vi "configurePerChannel.vi"(8 "error in (no error)":errorcluster, 10 "physical channels":string, 11 "K2602 in":refnum<class "K2602.lvclass">) -> (0 "error out":errorcluster, 3 "K2602 out":refnum<class "K2602.lvclass">)   [LabVIEW 2009, in "Hardware.lvlib" / "Channels.lvlib" / "K2602.lvclass"]
uses:
  K2602.lvclass
  K2602.lvclass/K2602.ctl
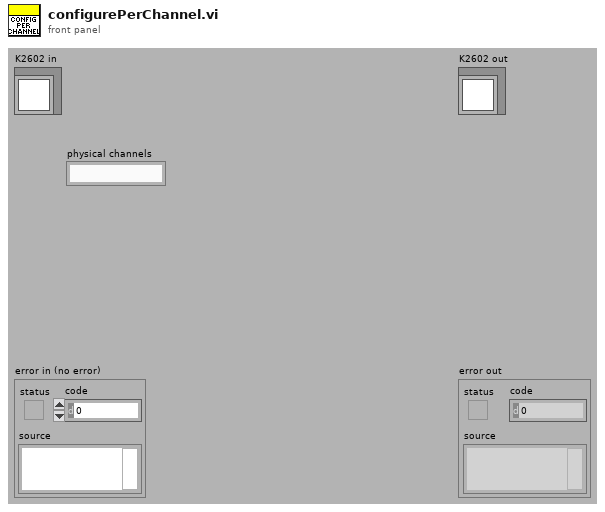
[diagram p1: front panel]
types:
  T1 = cluster{"Range":cluster{"current":dbl, "voltage":dbl}, "triggering_inUse":cluster{"start_trigger":string, "clock":string}, "Limits":cluster{"VoltageLimit":dbl, "CurrentLimit":dbl}}[]
  T2 = cluster{"Range":cluster{"current":dbl, "voltage":dbl}, "triggering_inUse":cluster{"start_trigger":string, "clock":string}, "Limits":cluster{"VoltageLimit":dbl, "CurrentLimit":dbl}}
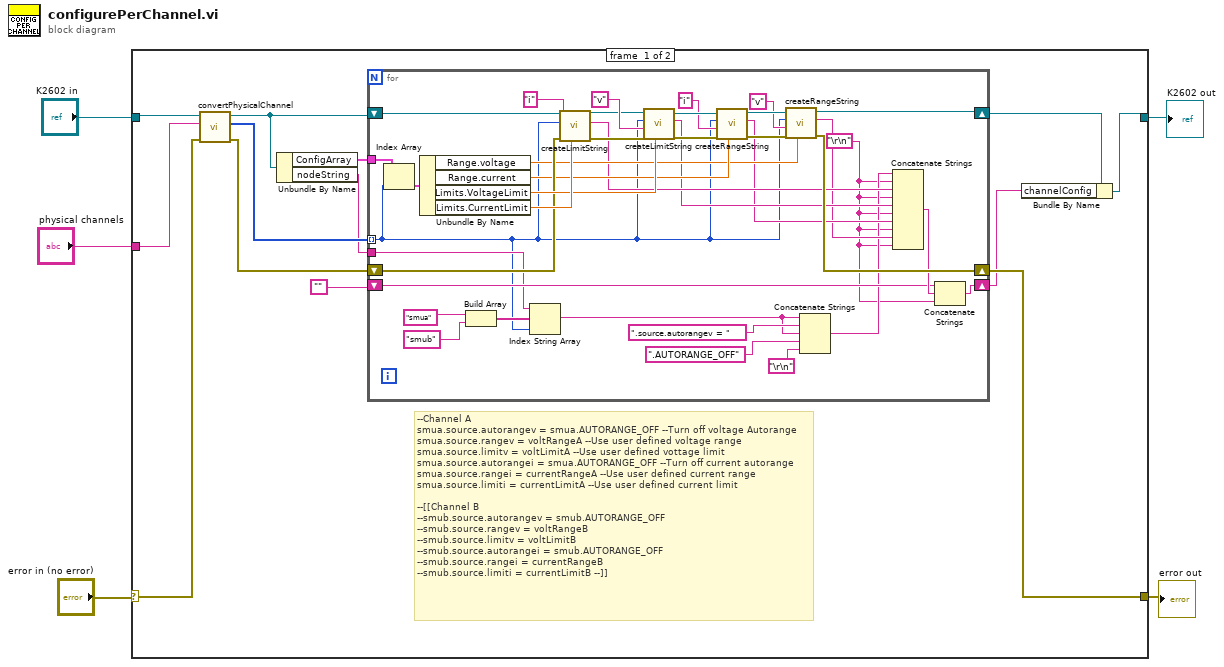
[diagram p0: block diagram]
diagram:
  n1 = case shown="No Error" "error in (no error)" {
    selector: "error in (no error)" -> [w16 w57]
    tunnel: "K2602 in" -> [w15 w58]
    tunnel: [w8 w58] -> w3
    tunnel: [w18 w57] -> w2
    tunnel: "physical channels" -> [w12 _]
    frame #0 {
      # "--Channel A\nsmua.source.autorangev = smua.AUTORANGE_OFF --Turn off voltage Autorange\nsmua.source.rangev = voltRangeA --Use user defined voltage range\nsmua.source.limitv = voltLimitA --Use user defined vottage limit\nsmua.source.autorangei = smua.AUTORANGE_OFF --Turn off current autorange\nsmua.source.rangei = currentRangeA --Use user defined current range\nsmua.source.limiti = currentLimitA --Use user defined current limit\n\n--[[Channel B\n--smub.source.autorangev = smub.AUTORANGE_OFF\n--smub.source.rangev = voltRangeB\n--smub.source.limitv = voltLimitB\n--smub.source.autorangei = smub.AUTORANGE_OFF\n--smub.source.rangei = currentRangeB\n--smub.source.limiti = currentLimitB --]]"
      n2 = call "convertPhysicalChannel.vi"("error in (no error)"=w16, "physicalChannels"=w12, "K2602 in"=w15) -> ("error out"=w17:errorcluster, "channel"=w13:i32[], "K2602 out"=w14:refnum<class "K2602.lvclass">)  [unwired: 6 in]
      n3 = Unbundle By Name(w14) -> ("ConfigArray"=w6:T1, "nodeString"=w7:string)
      n4 = for {
        shift-right: [w41] -> w9
        shift-left: w14 -> [w56]
        shift-right: [w39] -> w18
        shift-left: w17 -> [w49]
        tunnel: w13 -> [w20] mode=indexing
        shift-right: [w32] -> w10
        shift-left: "" -> [w33]
        tunnel: w7 -> [w22]
        tunnel: w6 -> [w21]
        w26 = "\r\n"
        n5 = Index Array(array=w21, index=w20) -> (element=w19:T2)
        n6 = Unbundle By Name(w19) -> ("Range.voltage"=w40:dbl, "Range.current"=w45:dbl, "Limits.VoltageLimit"=w50:dbl, "Limits.CurrentLimit"=w51:dbl)
        n7 = Build Array("smua", "smub") -> (w29:string[])
        n8 = Index String Array(1:w20, 2:w29, 3:w22) -> (0:w25:string)
        n9 = call "createLimitString.vi"("Limit (0.000)"=w51, "error in (no error)"=w49, "Function"="i", "Channel (Channel A)"=w20, "K2602 in"=w56) -> ("error out"=w52:errorcluster, "Limit string"=w38:string, "K2602 out"=w53:refnum<class "K2602.lvclass">)  [unwired: 4 in]
        n10 = call "createLimitString.vi"("Limit (0.000)"=w50, "error in (no error)"=w52, "Function"="v", "Channel (Channel A)"=w20, "K2602 in"=w53) -> ("error out"=w48:errorcluster, "Limit string"=w37:string, "K2602 out"=w47:refnum<class "K2602.lvclass">)  [unwired: 4 in]
        n11 = call "createRangeString.vi"("range (0.000)"=w45, "error in (no error)"=w48, "Function"="i", "Channel (Channel A)"=w20, "K2602 in"=w47) -> ("error out"=w44:errorcluster, "Limit string"=w36:string, "K2602 out"=w43:refnum<class "K2602.lvclass">)  [unwired: 4 in]
        n12 = call "createRangeString.vi"("range (0.000)"=w40, "error in (no error)"=w44, "Function"="v", "Channel (Channel A)"=w20, "K2602 in"=w43) -> ("error out"=w39:errorcluster, "Limit string"=w35:string, "K2602 out"=w41:refnum<class "K2602.lvclass">)  [unwired: 4 in]
        n13 = Concatenate Strings(w25, ".source.autorangev = ", w25, ".AUTORANGE_OFF", "\r\n") -> (w27:string)
        n14 = Concatenate Strings(w27, w26, w38, w26, w37, w26, w36, w26, w35, w26) -> (w34:string)
        n15 = Concatenate Strings(w33, w34, w26) -> (w32:string)
      }
      n16 = Bundle By Name(cluster=w9, "channelConfig"=w10) -> (w8:refnum<class "K2602.lvclass">)
    }
    frame #1 {
    }
  }
  "error out" <- w2
  "K2602 out" <- w3
